vi "Record Text.vi"(8 "error in (no error)":errorcluster, 10 "Slide Output path in":path, 11 "Slide Information in":T1) -> (0 "error out":errorcluster, 2 "Slide Output path out":path, 3 "Slide Information out":T1)   [LabVIEW 2015]
uses:
  Slide Info..cluster.ctl
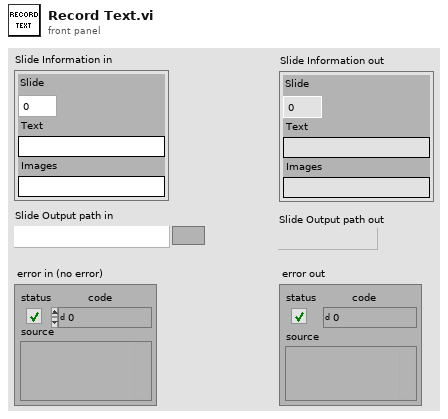
[diagram p1: front panel]
types:
  T1 = typedef "Slide Info..cluster.ctl" = cluster{"Slide":i32, "Text":string, "Images":string}
  T2 = enum16{"open", "replace", "create", "open or create", "replace or create", "replace or create with confirmation"}
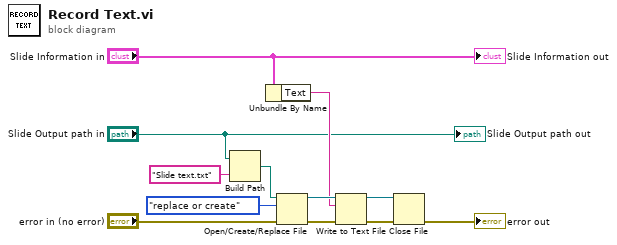
[diagram p0: block diagram]
diagram:
  n1 = Build Path(base path="Slide Output path in", name or relative path="Slide text.txt") -> (appended path=w5:path)
  n2 = Unbundle By Name("Slide Information in") -> ("Text"=w6:string)
  n3 = Open/Create/Replace File(file path (use dialog)=w5, error in="error in (no error)", operation (0:open)=T2."replace or create") -> (refnum out=w7:refnum<file>, error out=w10:errorcluster)  [unwired: 3 in, 1 out]
  n4 = Write to Text File(file (use dialog)=w7, text=w6, error in=w10) -> (refnum out=w1:refnum<file>, error out=w8:errorcluster)  [unwired: 1 in, 1 out]
  n5 = Close File(refnum=w1, error in=w8) -> (error out=→"error out":errorcluster)  [unwired: 1 out]
  "Slide Information out" <- "Slide Information in"
  "Slide Output path out" <- "Slide Output path in"
